vi "Update XY Graph Settings.vi"(10 "Persistent Data":T4 {"Graph Props"."Scale Properties"."X.Format" items=["Decimal", "Scientific", "Engineering", "Binary", "Octal", "Hexadecimal", "Relative Time", "Time and Date", "SI", "Automatic"]; "Graph Props"."Scale Properties"."Y.Precision:" items=["0", "1", "2", "3", "4", "5", "6", "7"]; "Graph Props"."Scale Properties"."Y.Format" items=["Decimal", "Scientific", "Engineering", "Binary", "Octal", "Hexadecimal", "Relative Time", "Time and Date", "SI", "Automatic"]; "Graph Props"."Scale Properties"."X.Precision" items=["0", "1", "2", "3", "4", "5", "6", "7"]}, 11 "Waveform Graph Data in":T1={"Custom Data"=variant, "EventRegs"={"SystemChange"=refnum, "WorkspaceState"=refnum, "Graph"=refnum, "Wks&Dialog&Periodic"=refnum}, "References"={"X.Scale.Auto"=refnum, "Y.Scale.Auto"=refnum, "X.Scale.Once"=refnum, "Y.Scale.Once"=refnum, "LegendVis"=refnum, "Graph"=refnum}, "Persistent Data"={"Label"="", "Graph Props"={"Plots"=[], "Legend:Number of Rows"=0, "Scale Properties"={"X.Auto"=FALSE, "X.Min"=0.0, "X.Max"=0.0, "X.IgnoreTS"=FALSE, "X.Precision"=0, "X.Label:"="", "X.LabelVis"=FALSE, "X.DefLabel"=FALSE, "Y.Auto"=FALSE, "Y.Min"=0.0, "Y.Max"=0.0, "Y.Format"=0, "Y.Precision:"=0, "Y.Label:"="", "Y.LabelVis"=FALSE, "Y.DefLabel"=FALSE, "X.Format"=0}, "Legend:Visible"=TRUE, "BgColor"=0, "Last Plot Width"=0, "Resize"=FALSE}, "UDP Data"={"Decimation"=0, "UDP Buffer Size"=0, "History Length"=0.0, "Update Rate"=enum."15 Hz", "Channel Paths"=[], "Channel Names"=[]}}, "System"={"To Workspace"=refnum, "From Workspace"=refnum, "NIVS helper"=refnum, "Gtwy"="", "Root"=refnum, "Workspace"=refnum, "SystemStateRefs"={"CustDatRef"=refnum, "EvtRef"=refnum, "Target State User Event"=refnum}, "Connected?"=FALSE, "FromDialog"=refnum, "ErrFlag"=FALSE, "New"=FALSE, "ErrState"="", "Save"=FALSE, "Hold"=FALSE, "Periodic"=refnum, "ToDialog"=refnum, "DialogEventReg"=refnum, "UseSavedWidth"=FALSE, "TreeBrowserEventReg"=refnum, "UDPChannelStreamSession"=refnum, "Valid Channels?"=FALSE, "Update Graph"=refnum, "UDP Queue"=refnum, "Graph Update Queue"=refnum}, "GraphData"=[], "UDP Stream Active?"=FALSE} {"Persistent Data"."Graph Props"."Scale Properties"."X.Format" items=["Decimal", "Scientific", "Engineering", "Binary", "Octal", "Hexadecimal", "Relative Time", "Time and Date", "SI", "Automatic"]; "Persistent Data"."Graph Props"."Scale Properties"."Y.Precision:" items=["0", "1", "2", "3", "4", "5", "6", "7"]; "Persistent Data"."Graph Props"."Scale Properties"."Y.Format" items=["Decimal", "Scientific", "Engineering", "Binary", "Octal", "Hexadecimal", "Relative Time", "Time and Date", "SI", "Automatic"]; "Persistent Data"."Graph Props"."Scale Properties"."X.Precision" items=["0", "1", "2", "3", "4", "5", "6", "7"]}) -> (2 "Waveform Graph Data out":T1={"Custom Data"=variant, "EventRegs"={"SystemChange"=refnum, "WorkspaceState"=refnum, "Graph"=refnum, "Wks&Dialog&Periodic"=refnum}, "References"={"X.Scale.Auto"=refnum, "Y.Scale.Auto"=refnum, "X.Scale.Once"=refnum, "Y.Scale.Once"=refnum, "LegendVis"=refnum, "Graph"=refnum}, "Persistent Data"={"Label"="", "Graph Props"={"Plots"=[], "Legend:Number of Rows"=0, "Scale Properties"={"X.Auto"=FALSE, "X.Min"=0.0, "X.Max"=0.0, "X.IgnoreTS"=FALSE, "X.Precision"=0, "X.Label:"="", "X.LabelVis"=FALSE, "X.DefLabel"=FALSE, "Y.Auto"=FALSE, "Y.Min"=0.0, "Y.Max"=0.0, "Y.Format"=0, "Y.Precision:"=0, "Y.Label:"="", "Y.LabelVis"=FALSE, "Y.DefLabel"=FALSE, "X.Format"=0}, "Legend:Visible"=TRUE, "BgColor"=0, "Last Plot Width"=0, "Resize"=FALSE}, "UDP Data"={"Decimation"=0, "UDP Buffer Size"=0, "History Length"=0.0, "Update Rate"=enum."15 Hz", "Channel Paths"=[], "Channel Names"=[]}}, "System"={"To Workspace"=refnum, "From Workspace"=refnum, "NIVS helper"=refnum, "Gtwy"="", "Root"=refnum, "Workspace"=refnum, "SystemStateRefs"={"CustDatRef"=refnum, "EvtRef"=refnum, "Target State User Event"=refnum}, "Connected?"=FALSE, "FromDialog"=refnum, "ErrFlag"=FALSE, "New"=FALSE, "ErrState"="", "Save"=FALSE, "Hold"=FALSE, "Periodic"=refnum, "ToDialog"=refnum, "DialogEventReg"=refnum, "UseSavedWidth"=FALSE, "TreeBrowserEventReg"=refnum, "UDPChannelStreamSession"=refnum, "Valid Channels?"=FALSE, "Update Graph"=refnum, "UDP Queue"=refnum, "Graph Update Queue"=refnum}, "GraphData"=[], "UDP Stream Active?"=FALSE} {"Persistent Data"."Graph Props"."Scale Properties"."X.Format" items=["Decimal", "Scientific", "Engineering", "Binary", "Octal", "Hexadecimal", "Relative Time", "Time and Date", "SI", "Automatic"]; "Persistent Data"."Graph Props"."Scale Properties"."Y.Precision:" items=["0", "1", "2", "3", "4", "5", "6", "7"]; "Persistent Data"."Graph Props"."Scale Properties"."Y.Format" items=["Decimal", "Scientific", "Engineering", "Binary", "Octal", "Hexadecimal", "Relative Time", "Time and Date", "SI", "Automatic"]; "Persistent Data"."Graph Props"."Scale Properties"."X.Precision" items=["0", "1", "2", "3", "4", "5", "6", "7"]}, 3 "State Array":string[](array[string]))   [LabVIEW 2020, in "Workspace MultiY Graph.lvlib"]
uses:
  Workspace MultiY Graph.lvlib
  XY Persistent Data.ctl
  XY Graph Properties.ctl
  XY Plot Properties.ctl
  XY Scale Properties.ctl
  XY Scale Precision.ctl
  XY Scale Format.ctl
  UDP Data.ctl
  Update Rate.ctl
  XY Top level workspace graph data.ctl
  <vilib>/NI VeriStand/Execution/Workspace/SystemStateRegEventRef.ctl
  <vilib>/NI VeriStand/Execution/Workspace/Target State Info.ctl
  <vilib>/NI VeriStand/Execution/Workspace/Target State.ctl
  <vilib>/NI VeriStand/Display Template Support/DisplayTemplateSupport.llb/enum_Display Template Handler Minimal To Widget Msg.ctl
  XY Dialog Msg to Control.ctl
  XY Dialog Msg Type.ctl
  XY References.ctl
  <vilib>/NI VeriStand/Display Template Support/DisplayTemplateSupport.llb/enum_Display Template Handler Minimal To Workspace.ctl
  NationalInstruments.VeriStand.SystemStorage
  <vilib>/NI VeriStand/Execution/Workspace/WorkspaceAPI.ctl
  NationalInstruments.VeriStand.ClientAPI
  <vilib>/NI VeriStand/Execution/Workspace/SystemStateEventRef.ctl
  XY Control Msg to Dialog.ctl
  <vilib>/NI VeriStand/UI Controls/Tree and Alias Browser/Net Event Data Ref.ctl
  <vilib>/NI VeriStand/UI Controls/Tree and Alias Browser/Net Event Data.ctl
  <vilib>/NI VeriStand/UI Controls/Tree and Alias Browser/Net Event.ctl
  <vilib>/NI VeriStand/Execution/Workspace/UDPChannelStreamSession.ctl
  UDP Queue Data.ctl
  UDP Action State.ctl
  Graph Update Queue Data.ctl
  Graph Update Action State.ctl
  <vilib>/NI VeriStand/Execution/Workspace/NI_VS Workspace ExecutionAPI.lvlib
  <vilib>/NI VeriStand/UI Controls/Tree and Alias Browser/NI_VS UI Tree Alias Browser.lvlib
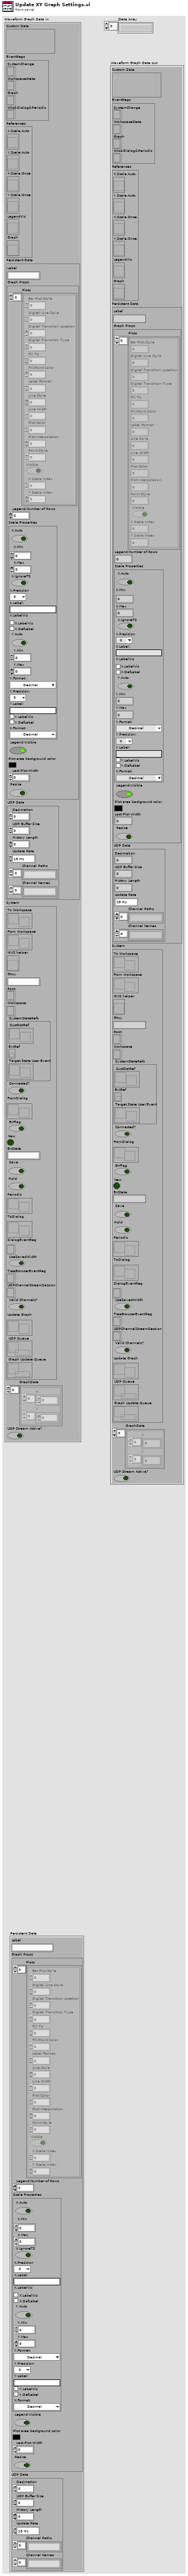
[diagram p1: front panel]
types:
  T1 = typedef "Workspace MultiY Graph.lvlib/XY Top level workspace graph data.ctl" = cluster{"Custom Data":variant, "EventRegs":cluster{"SystemChange":T2, "WorkspaceState":refnum<event-registration>, "Graph":refnum<event-registration>, "Wks&Dialog&Periodic":refnum<event-registration>}, "References":T3, "Persistent Data":T4, "System":cluster{"To Workspace":refnum<user-event>, "From Workspace":refnum<user-event>, "NIVS helper":refnum<vi>, "Gtwy":string, "Root":refnum<k24>, "Workspace":T12, "SystemStateRefs":T13, "Connected?":bool, "FromDialog":refnum<user-event>, "ErrFlag":bool, "New":bool, "ErrState":string, "Save":bool, "Hold":bool, "Periodic":refnum<user-event>, "ToDialog":refnum<user-event>, "DialogEventReg":refnum<event-registration>, "UseSavedWidth":bool, "TreeBrowserEventReg":refnum<event-registration>, "UDPChannelStreamSession":T14, "Valid Channels?":bool, "Update Graph":refnum<user-event>, "UDP Queue":refnum<queue>, "Graph Update Queue":refnum<queue>}, "GraphData":cluster{"X":dbl[], "Y":dbl[]}[], "UDP Stream Active?":bool}
  T2 = typedef "NI_VS Workspace ExecutionAPI.lvlib/SystemStateRegEventRef.ctl" = refnum<event-registration>
  T3 = typedef "Workspace MultiY Graph.lvlib/XY References.ctl" = cluster{"X.Scale.Auto":refnum<vi>, "Y.Scale.Auto":refnum<vi>, "X.Scale.Once":refnum<vi>, "Y.Scale.Once":refnum<vi>, "LegendVis":refnum<vi>, "Graph":refnum<vi>}
  T4 = typedef "Workspace MultiY Graph.lvlib/XY Persistent Data.ctl" = cluster{"Label":string, "Graph Props":T5, "UDP Data":T10}
  T5 = typedef "Workspace MultiY Graph.lvlib/XY Graph Properties.ctl" = cluster{"Plots":T6[], "Legend:Number of Rows":u32, "Scale Properties":T7, "Legend:Visible":bool, "BgColor":u32, "Last Plot Width":u32, "Resize":bool}
  T6 = typedef "Workspace MultiY Graph.lvlib/XY Plot Properties.ctl" = cluster{"Bar Plot Style":u8, "Digital Line Style":u8, "Digital Transition Location":u8, "Digital Transition Type":u8, "Fill To":i16, "Fill/Point Color":u32, "Label Format":u8, "Line Style":u8, "Line Width":u8, "Plot Color":u32, "Plot Interpolation":u8, "Point Style":u8, "Visible":bool, "X Scale Index":u32, "Y Scale Index":u32}
  T7 = typedef "Workspace MultiY Graph.lvlib/XY Scale Properties.ctl" = cluster{"X.Auto":bool, "X.Min":dbl, "X.Max":dbl, "X.IgnoreTS":bool, "X.Precision":T8, "X.Label:":string, "X.LabelVis":bool, "X.DefLabel":bool, "Y.Auto":bool, "Y.Min":dbl, "Y.Max":dbl, "Y.Format":T9, "Y.Precision:":T8, "Y.Label:":string, "Y.LabelVis":bool, "Y.DefLabel":bool, "X.Format":T9}
  T8 = typedef "Workspace MultiY Graph.lvlib/XY Scale Precision.ctl" = u8
  T9 = typedef "Workspace MultiY Graph.lvlib/XY Scale Format.ctl" = u8
  T10 = typedef "Workspace MultiY Graph.lvlib/UDP Data.ctl" = cluster{"Decimation":i32, "UDP Buffer Size":u32, "History Length":dbl, "Update Rate":T11, "Channel Paths":string[], "Channel Names":string[]}
  T11 = typedef "Workspace MultiY Graph.lvlib/Update Rate.ctl" = enum8{"15 Hz", "10 Hz", "5 Hz", "4 Hz", "3 Hz", "2 Hz", "1 Hz", "0.5 Hz"}
  T12 = typedef "NI_VS Workspace ExecutionAPI.lvlib/WorkspaceAPI.ctl" = refnum<k24>
  T13 = typedef "NI_VS Workspace ExecutionAPI.lvlib/SystemStateEventRef.ctl" = cluster{"CustDatRef":refnum<user-event>, "EvtRef":refnum<k27>, "Target State User Event":refnum<user-event>}
  T14 = typedef "NI_VS Workspace ExecutionAPI.lvlib/UDPChannelStreamSession.ctl" = refnum<k24>
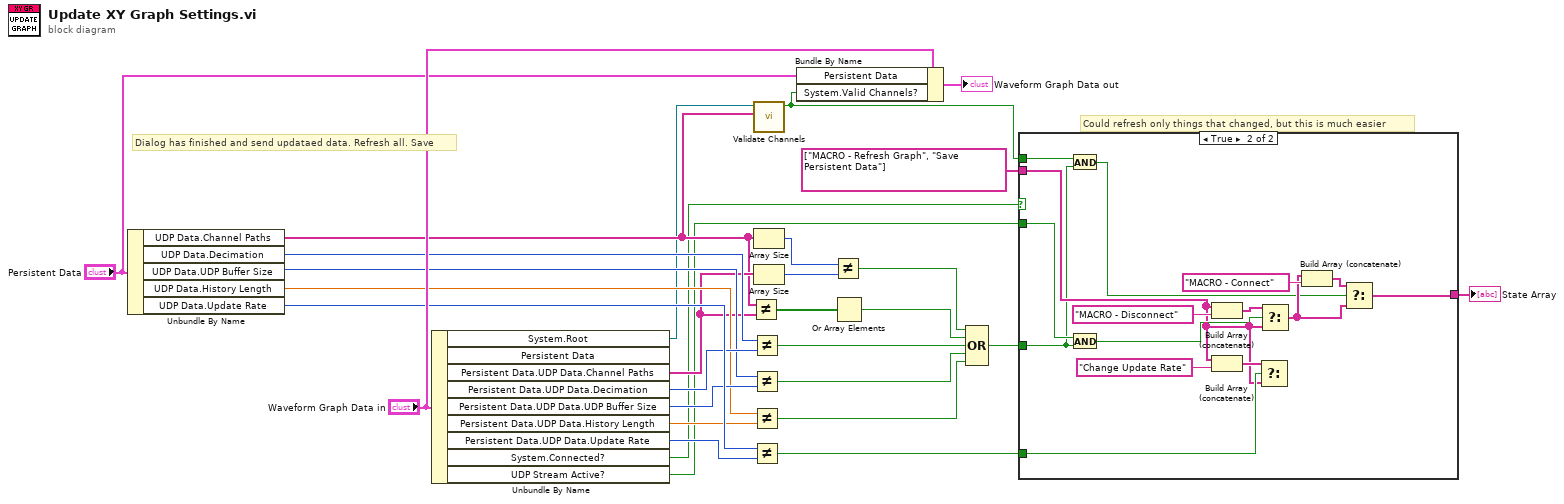
[diagram p0: block diagram]
diagram:
  # "Could refresh only things that changed, but this is much easier"
  # "Dialog has finished and send updataed data. Refresh all. Save"
  n1 = Unbundle By Name("Persistent Data") -> ("UDP Data.Channel Paths"=w5:string[], "UDP Data.Decimation"=w20:i32, "UDP Data.UDP Buffer Size"=w18:u32, "UDP Data.History Length"=w17:dbl, "UDP Data.Update Rate"=w24:T11)
  n2 = Unbundle By Name("Waveform Graph Data in") -> ("System.Root"=w3:refnum<k24>, "Persistent Data.UDP Data.Channel Paths"=w9:string[], "Persistent Data.UDP Data.Decimation"=w21:i32, "Persistent Data.UDP Data.UDP Buffer Size"=w19:u32, "Persistent Data.UDP Data.History Length"=w16:dbl, "Persistent Data.UDP Data.Update Rate"=w25:T11, "System.Connected?"=w1:bool, "UDP Stream Active?"=w2:bool)  [unwired: 1 out]
  n3 = Not Equal?(x=w5, y=w9) -> (x != y?=w22:bool[])
  n4 = Not Equal?(x=w20, y=w21) -> (x != y?=w15:bool)
  n5 = Not Equal?(x=w18, y=w19) -> (x != y?=w14:bool)
  n6 = Not Equal?(x=w17, y=w16) -> (x != y?=w13:bool)
  n7 = Not Equal?(x=w24, y=w25) -> (x != y?=w7:bool)
  n8 = call "Validate Channels.vi"("Channel Paths"=w5, "Root"=w3) -> ("Valid Channels?"=w4:bool)  [unwired: 9 in]
  n9 = Array Size(array=w5) -> (size(s)=w11:i32)
  n10 = Array Size(array=w9) -> (size(s)=w10:i32)
  n11 = Bundle By Name(cluster="Waveform Graph Data in", "Persistent Data"="Persistent Data", "System.Valid Channels?"=w4) -> (→"Waveform Graph Data out":T1)
  n12 = Not Equal?(x=w11, y=w10) -> (x != y?=w8:bool)
  n13 = Or Array Elements(Boolean array=w22) -> (logical OR=w12:bool)
  n14 = Compound Arithmetic op=OR(w8, w12, w15, w14, w13) -> (w6:bool)
  n15 = case shown="True" w1 {
    tunnel: string[] ["MACRO - Refresh Graph", "Save Persistent Data"] -> [w30 w34]
    tunnel: [w30 w35] -> w29
    tunnel: w2 -> [_ w42]
    tunnel: w7 -> [_ w45]
    tunnel: w6 -> [_ w33]
    tunnel: w4 -> [_ w32]
    frame False {
    }
    frame True {
      n16 = And(x=w32, y=w33) -> (x .and. y?=w31:bool)
      n17 = And(x=w42, y=w33) -> (x .and. y?=w41:bool)
      n18 = Build Array (concatenate)(w34, "MACRO - Disconnect") -> (w39:string[])
      n19 = Build Array (concatenate)(w34, "Change Update Rate" ("f")) -> (w43:string[])
      n20 = Select(t=w43, s=w45, f=w34) -> ()  [unwired: 1 out]
      n21 = Select(t=w39, s=w41, f=w34) -> (s? t:f=w36:string[])
      n22 = Build Array (concatenate)(w36, "MACRO - Connect") -> (w38:string[])
      n23 = Select(t=w38, s=w31, f=w36) -> (s? t:f=w35:string[])
    }
  }
  "State Array" <- w29
